vi "countdown.vi"(11 "countdown time\n(sec)":dbl=5.0) -> ()   [LabVIEW 2017]
uses:
  <vilib>/Utility/miscctls.llb/LVPointTypeDef.ctl
  <vilib>/Platform/TimedLoop/XDataNode/timing_clust.ctl
  <vilib>/Platform/TimedLoop/XDataNode/nitl_modes.ctl
  <vilib>/Platform/TimedLoop/XDataNode/wakeup.ctl
  <vilib>/Platform/TimedLoop/XDataNode/XDataNode.xnode
  <vilib>/Platform/TimedLoop/XDataNode/XDNodeRunTimeDep.lvlib
panel:
  out "resulting string":string
types:
  T1 = typedef "LVPointTypeDef.ctl" = cluster{"Horizontal":i16, "Vertical":i16}
  T2 = typedef "XDNodeRunTimeDep.lvlib/timing_clust.ctl" = cluster{"Expected End [f-1]":u64, "Actual End [f-1]":u64, "Finished Late? [f-1]":bool, "Expected End [i-1]":u64, "Actual End [i-1]":u64, "Finished Late? [i-1]":bool, "Expected Start [i]":u64, "Actual Start [i]":u64, "Expected Start [f]":u64, "Actual Start [f]":u64, "Source Name":string, "Structure Name":string, "Period":i64, "Deadline":i64, "Offset":i64, "Start":i64, "Priority":i32, "Timeout":i32, "Mode":T3, "Wakeup Reason":T4, "Error":errorcluster, "Source Type":string, "Secondary Source Type":string, "Global End Time":u64, "Global Start Time":u64, "Frame Duration":u64, "Iteration Duration":u64, "Assigned CPU":i32, "I/O Scan Engine Mode":u32}
  T3 = typedef "XDNodeRunTimeDep.lvlib/nitl_modes.ctl" = enum32{"No Change", "Process missed periods, maintain original phase", "Discard missed periods, maintain original phase", "Process missed periods, ignore original phase", "Discard missed periods, ignore original phase"}
  T4 = typedef "XDNodeRunTimeDep.lvlib/wakeup.ctl" = enum32{"Normal", "Aborted", "Asynchronous wakeup", "Timing source error", "Timed loop error", "Timeout"}
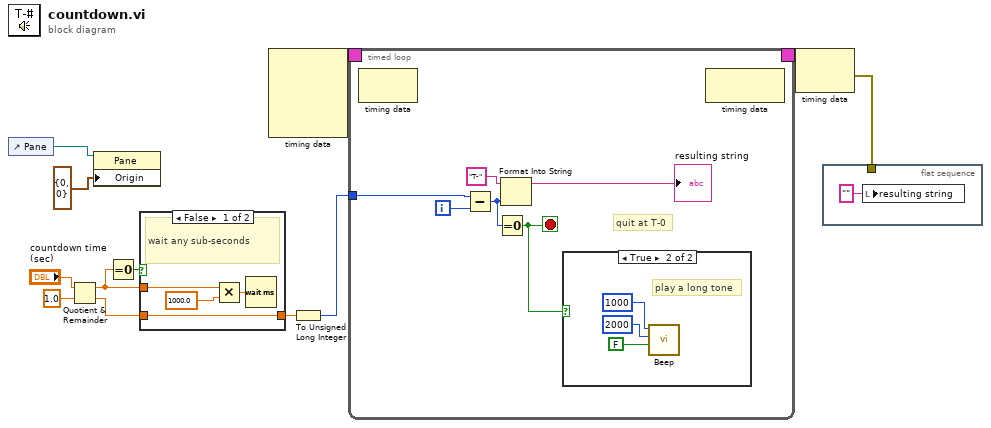
[diagram p0: block diagram]
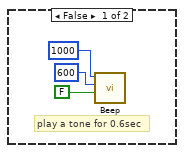
[diagram p3: hidden frame]
diagram:
  n1 = control-ref of="Pane"() -> (w2:refnum<vi>)
  n2 = Quotient & Remainder(x="countdown time\n(sec)", y=1.0) -> (x-y*floor(x/y)=w8:dbl, floor(x/y)=w6:dbl)
  n3 = property class="Pane"(reference=w2, "Origin"=T1 {"Horizontal"=0, "Vertical"=0}) -> ()  [unwired: 1 in, 2 out]
  n4 = Equal To 0?(x=w8) -> (x = 0?=w7:bool)
  n5 = case shown="False" w7 {
    tunnel: w8 -> [w14 _]
    tunnel: w6 -> [w16 w17]
    tunnel: [w16 w17] -> w5
    frame False {
      # "wait any sub-seconds"
      n6 = Multiply(x=w14, y=1000.0) -> (x*y=w15:dbl)
      n7 = Wait (ms)(milliseconds to wait=w15) -> ()  [unwired: 1 out]
    }
    frame True {
      # "perfect integer"
    }
  }
  n8 = node-c288() -> (w12:T2)  [unwired: 4 in]
  n9 = To Unsigned Long Integer(number=w5) -> (unsigned 32bit integer=w4:u32)
  n10 = timed-loop {
    timing: w12 -> [_]
    timing-out: [_] -> w11
    tunnel: w4 -> [w19]
    i -> [w22]
    stop <- w20 stop-if-true
    # "quit at T-0"
    n11 = node-c288() -> ()  [unwired: 1 in, 1 out]
    n12 = Subtract(x=w19, y=w22) -> (x-y=w21:u32)
    n13 = Equal To 0?(x=w21) -> (x = 0?=w20:bool)
    n14 = Format Into String(initial string="T-", w21) -> (resulting string=→"resulting string":string)  [unwired: 2 in, 1 out]
    n15 = case shown="True" w20 {
      frame False {
        # "play a tone for 0.6sec"
        n16 = call <vilib>:"Beep.vi"("use system alert? (T)"=FALSE, "duration (msec)"=u32 600, "frequency (Hz)"=u32 1000) -> ()  [unwired: 9 in]
      }
      frame True {
        # "play a long tone"
        n17 = call <vilib>:"Beep.vi"("use system alert? (T)"=FALSE, "duration (msec)"=u32 2000, "frequency (Hz)"=u32 1000) -> ()  [unwired: 9 in]
      }
    }
    n18 = node-c288() -> ()  [unwired: 1 in, 1 out]
  }
  n19 = node-c288(w11) -> (w1:errorcluster)
  n20 = flat-sequence {
    tunnel: w1 -> [_]
    frame #0 {
      n21 = local write "resulting string"("" ("resulting string")) -> ()
    }
  }
